vi "Set RTS and DTR states return CTS.vi"(7 "Assert DTR?":bool, 8 "error in (no error)":errorcluster, 9 "Assert RTS?":bool, 10 "Is serial open? (y)":bool=TRUE, 11 "VISA Refnum in":refnum<visa-resource-name>="COM30") -> (0 "error out":errorcluster, 2 "CTS asserted?":bool, 3 "Visa ref out":refnum<visa-resource-name>)   [LabVIEW 2013]
panel:
  out "Serial Settings:Modem Line Settings:Line RTS State":i16(ring)=-1 items=["Unknown"=-1, "Unasserted"=0, "Asserted"=1]
  out "Serial Settings:Modem Line Settings:Line DTR State":i16(ring)=-1 items=["Unknown"=-1, "Unasserted"=0, "Asserted"=1]
  out "Serial Settings:Modem Line Settings:Line CTS State":i16(ring)=-1 items=["Unknown"=-1, "Unasserted"=0, "Asserted"=1]
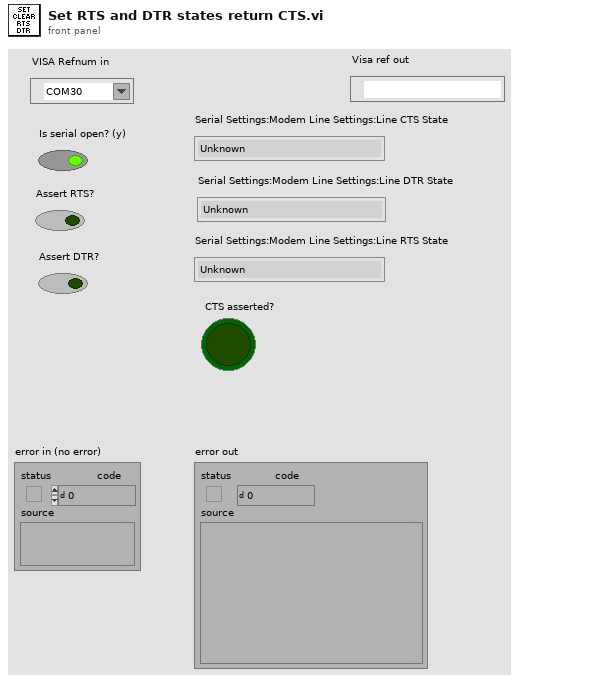
[diagram p1: front panel]
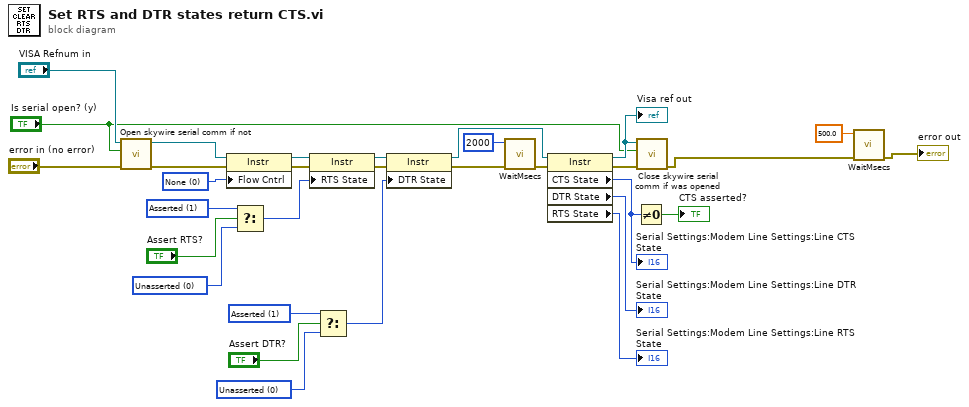
[diagram p0: block diagram]
diagram:
  w20 = i16 1 items=["Unknown"=-1, "Unasserted"=0, "Asserted"=1] ("Serial Settings:Modem Line Settings:Line DTR State")
  w21 = i16 0 items=["Unknown"=-1, "Unasserted"=0, "Asserted"=1] ("Serial Settings:Modem Line Settings:Line DTR State")
  w28 = i16 1 items=["Unknown"=-1, "Unasserted"=0, "Asserted"=1] ("Serial Settings:Modem Line Settings:Line DTR State")
  w27 = i16 0 items=["Unknown"=-1, "Unasserted"=0, "Asserted"=1] ("Serial Settings:Modem Line Settings:Line DTR State")
  w29 = u16 0 items=["None", "XON/XOFF", "RTS/CTS", "XON/XOFF & RTS/CTS", "DTR/DSR", "XON/XOFF & DTR/DSR"] ("Serial Settings:Flow Control")
  n1 = call "Open skywire serial comm if not.vi"("error in (no error)"="error in (no error)", "Is serial open?"="Is serial open? (y)", "VISA Refnum in"="VISA Refnum in") -> ("error out"=w12:errorcluster, "VISA Refnum out"=w13:refnum<visa-resource-name>)  [unwired: 7 in]
  n2 = property class="Instr"(reference=w13, error in=w12, "Flow Cntrl"=w29) -> (reference out=w24:refnum<visa-resource-name>, error out=w25:errorcluster)
  n3 = Select(t=w28, s="Assert RTS?", f=w27) -> (s? t:f=w26:i16)
  n4 = property class="Instr"(reference=w24, error in=w25, "RTS State"=w26) -> (reference out=w23:refnum<visa-resource-name>, error out=w22:errorcluster)
  n5 = Select(t=w20, s="Assert DTR?", f=w21) -> (s? t:f=w19:i16)
  n6 = property class="Instr"(reference=w23, error in=w22, "DTR State"=w19) -> (reference out=w14:refnum<visa-resource-name>, error out=w8:errorcluster)
  n7 = call "WaitMsecs.vi"("error in (no error)"=w8, "Wait Msecs"=u32 2000) -> ("error out"=w6:errorcluster)  [unwired: 9 in]
  n8 = property class="Instr"(reference=w14, error in=w6) -> (reference out=w11:refnum<visa-resource-name>, error out=w10:errorcluster, "CTS State"=w5:i16, "DTR State"=→"Serial Settings:Modem Line Settings:Line DTR State":i16, "RTS State"=→"Serial Settings:Modem Line Settings:Line RTS State":i16)
  "Serial Settings:Modem Line Settings:Line CTS State" <- w5
  "Visa ref out" <- w11
  n9 = Not Equal To 0?(x=w5) -> (x != 0?=→"CTS asserted?":bool)
  n10 = call "Close skywire serial comm if was opened.vi"("error in (no error)"=w10, "Is serial open?"="Is serial open? (y)", "VISA Refnum in"=w11) -> ("error out"=w2:errorcluster)  [unwired: 7 in, 1 out]
  n11 = call "WaitMsecs.vi"("error in (no error)"=w2, "Wait Msecs"=500.0) -> ("error out"=→"error out":errorcluster)  [unwired: 9 in]
